vi "Number to ASCII Code Array.vi"(10 "Numbet to transform":dbl format="%#_8g") -> (1 "Array - String":string[](array[string]), 2 "Array of ASCII Codes":u8[](array[numeric]))   [LabVIEW 2016]
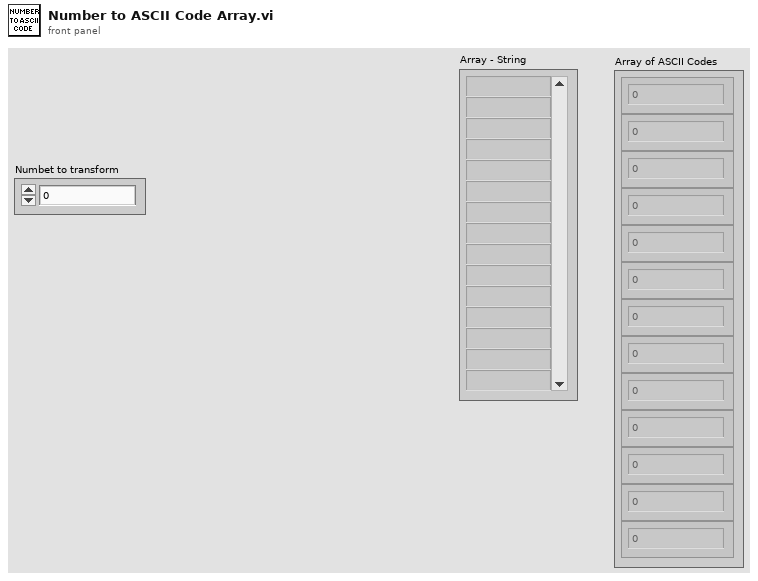
[diagram p1: front panel]
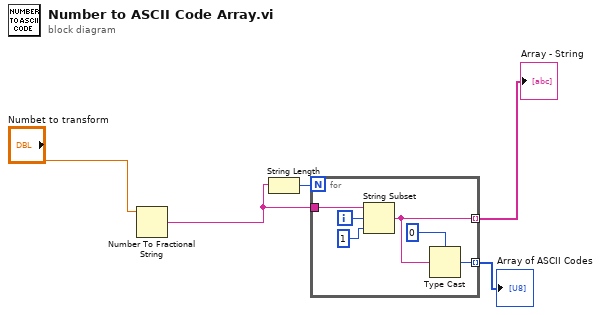
[diagram p0: block diagram]
diagram:
  n1 = Number To Fractional String(number="Numbet to transform") -> (F-format string=w4:string)  [unwired: 3 in]
  n2 = String Length(string=w4) -> (length=w5:i32)
  n3 = for {
    N: w5 -> [_]
    tunnel: w4 -> [w11]
    tunnel: [w7] -> w1 mode=indexing
    tunnel: [w6] -> w2 mode=indexing
    i -> [w10]
    n4 = String Subset(string=w11, offset (0)=w10, length (rest)=1 ("length (rest)")) -> (substring=w7:string)
    n5 = Type Cast(type=u8 0, x=w7) -> (*(type *) &x=w6:u8)
  }
  "Array of ASCII Codes" <- w2
  "Array - String" <- w1
